vi "draw box imaq.vi"(8 "Color":u32(colorbox)=16711680, 9 "error in (no error)":errorcluster, 10 "Rectangle":T2, 11 "image in":T1) -> (0 "error out":errorcluster, 3 "image out":T1)   [LabVIEW 2013]
uses:
  <vilib>/vision/Image Controls.llb/IMAQ Image.ctl
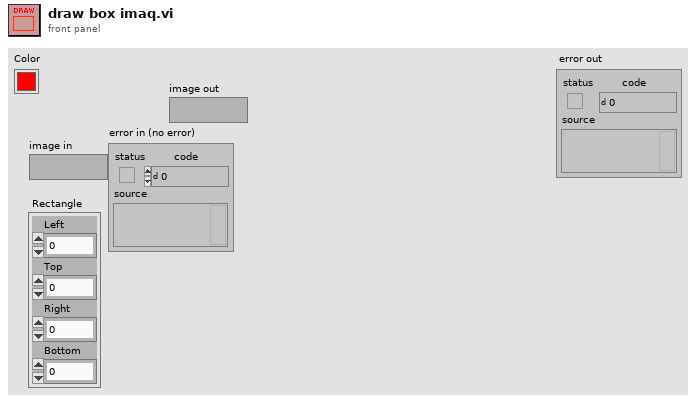
[diagram p1: front panel]
types:
  T1 = typedef "IMAQ Image.ctl" = refnum<image>
  T2 = cluster{"Left":i32, "Top":i32, "Right":i32, "Bottom":i32}
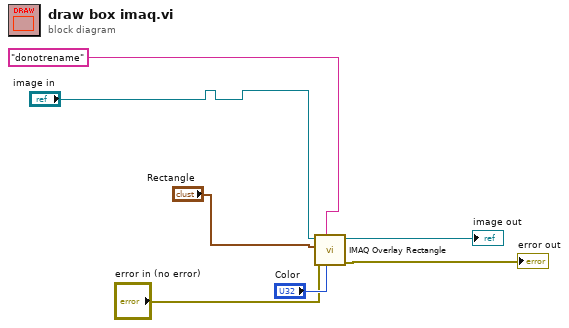
[diagram p0: block diagram]
diagram:
  n1 = call "IMAQ Overlay Rectangle"("Color"="Color", "Group"="donotrename" ("String"), "error in (no error)"="error in (no error)", "Rectangle"="Rectangle", "Image"="image in") -> ("error out"=→"error out":errorcluster, "Image Out"=→"image out":T1)  [unwired: 5 in]
